vi "InitDecorations.vi"   [LabVIEW 2019]
doc: "This VI initializes devices related directly to the decorations."
uses:
  <vilib>/Rock Robotics/SystemInterfaces/DIO/FPGA_DIOPWMChannel.ctl
  refnums.vi
types:
  T1 = typedef "FPGA_DIOPWMChannel.ctl" = enum8{"PWM 0", "PWM 1", "PWM 2", "PWM 3", "PWM 4", "PWM 5", "PWM 6", "PWM 7", "PWM 8", "PWM 9", "PWM MXP 0", "PWM MXP 1", "PWM MXP 2", "PWM MXP 3", "PWM MXP 4", "PWM MXP 5", "PWM MXP 6", "PWM MXP 7", "PWM MXP 8", "PWM MXP 9", "Invalid"}
  T2 = typedef "WPI_PWMDeviceRef.ctl" = cluster{"DeviceStatus":errorcluster, "PWM Channel":T1}
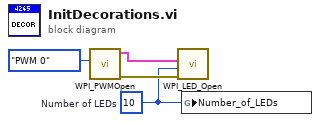
[diagram p0: block diagram]
diagram:
  w1 = u16 10  # Number of LEDs
  n1 = call <vilib>:"WPI_PWMOpen.vi"("PWM Channel"=FPGA_DIOPWMChannel."PWM 0") -> ("error out"=w3:errorcluster, "PWMDeviceRef"=w4:T2)  [unwired: 9 in]
  n2 = call <vilib>:"WPI_LED_Open.vi"("error in"=w3, "String Length"=w1, "PWMDeviceRef"=w4) -> ()  [unwired: 8 in, 1 out]
  n3 = global write "refnums.vi" "Number_of_LEDs"(w1) -> ()
